vi "Preferences.vi"() -> ()   [LabVIEW 2014]
uses:
  globals/AzCamGlobals.vi
panel:
  in  "Enable Telescope":bool
  in  "Enable Instrument":bool
  in  "ShowClientCommands":bool caption="Show client commands"
  in  "SequenceFlushing":enum32{"All", "Once", "None"}(radio)
  in  "Sequence\nDelay (secs)":dbl format="%#.3g"
  in  "ReadTemps":bool caption="Read temperatures"
  in  "Reload":bool
  in  "AutoTitle":bool caption="Auto title images"
  in  "ShowUserWarnings":bool=TRUE caption="Show User Warnings"
  in  "Use Sound":bool
  in  "Prompt4Title":bool caption="Prompt for Image Title"
  in  "ClearArray":bool=TRUE caption="Clear Array before each exposure"
  in  "Display image":bool=TRUE
  in  "Image Header File":path=path "NONE"
  in  "EditHeaderFile":bool
  in  "Exit":bool
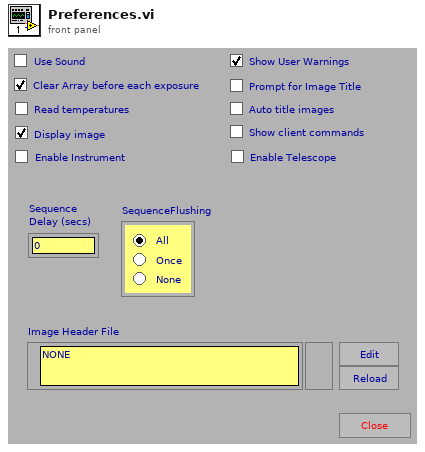
[diagram p1: front panel]
types:
  T1 = enum16{"Status", "CamTemp", "DewTemp", "GetExpose", "GetSequence", "SetExpose", "Filename", "ColBin", "RowBin"}
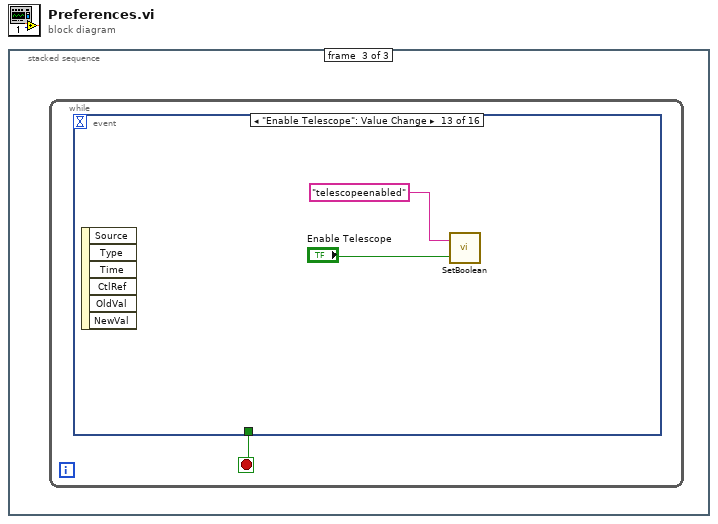
[diagram p0: block diagram]
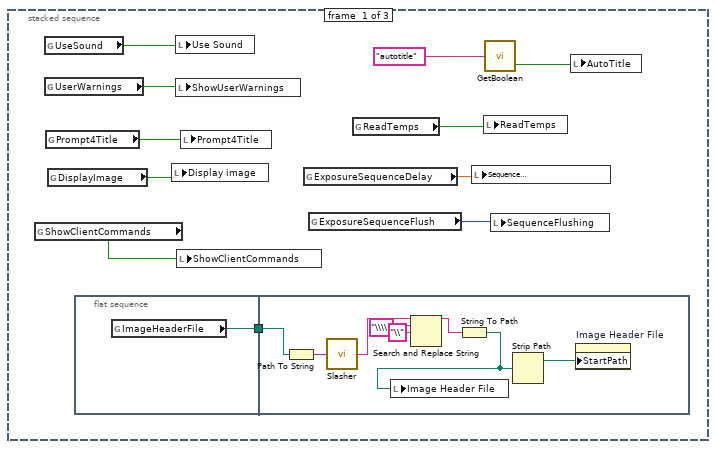
[diagram p2: hidden frame]
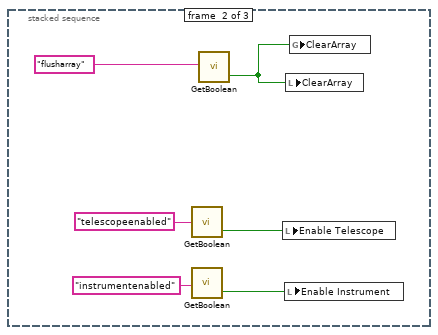
[diagram p3: hidden frame]
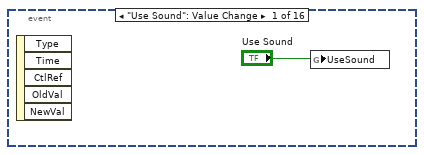
[diagram p4: hidden frame]
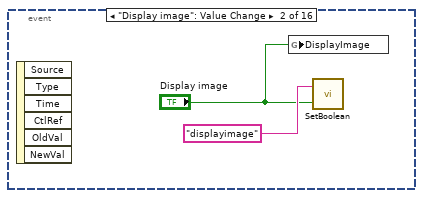
[diagram p5: hidden frame]
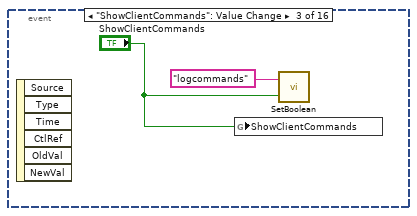
[diagram p6: hidden frame]
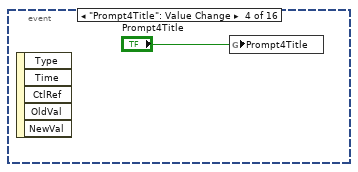
[diagram p7: hidden frame]
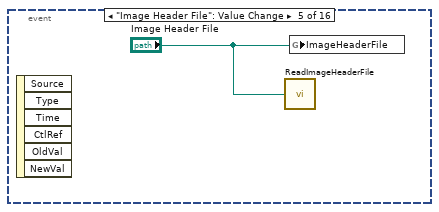
[diagram p8: hidden frame]
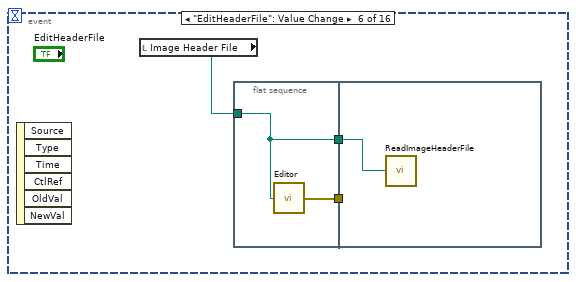
[diagram p9: hidden frame]
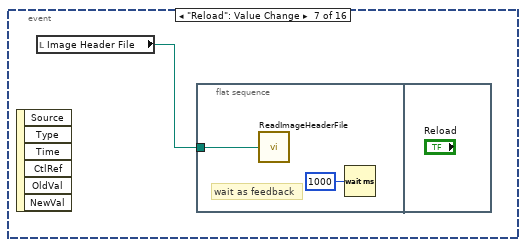
[diagram p10: hidden frame]
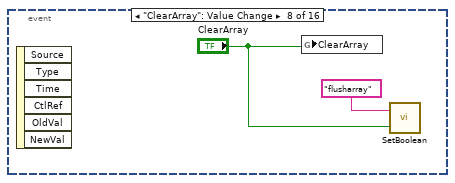
[diagram p11: hidden frame]
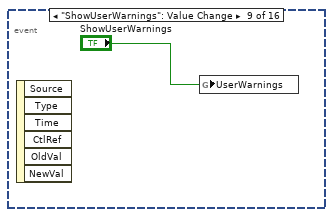
[diagram p12: hidden frame]
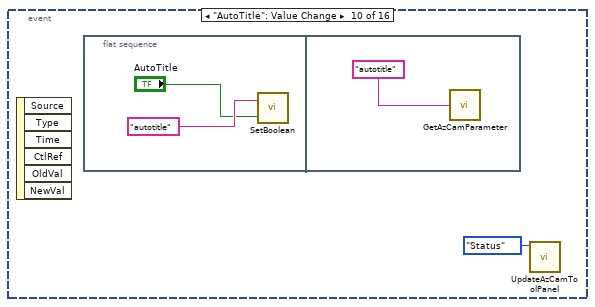
[diagram p13: hidden frame]
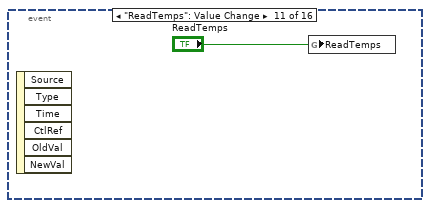
[diagram p14: hidden frame]
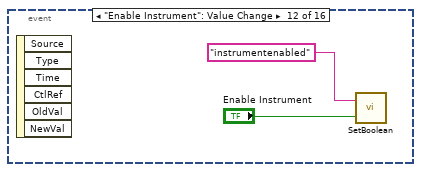
[diagram p15: hidden frame]
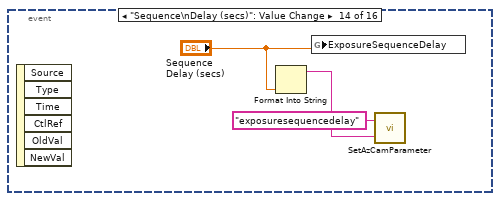
[diagram p16: hidden frame]
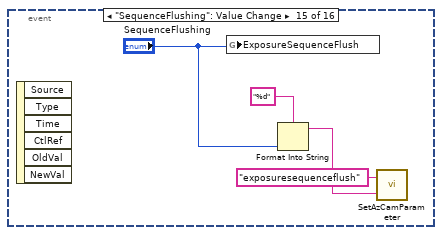
[diagram p17: hidden frame]
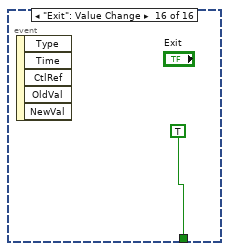
[diagram p18: hidden frame]
diagram:
  n1 = stacked-sequence {
    frame #0 {
      n2 = global read "AzCamGlobals.vi" "ShowClientCommands"() -> (w1:bool)
      n3 = global read "AzCamGlobals.vi" "UseSound"() -> (w7:bool)
      n4 = global read "AzCamGlobals.vi" "UserWarnings"() -> (w10:bool)
      n5 = global read "AzCamGlobals.vi" "Prompt4Title"() -> (w11:bool)
      n6 = global read "AzCamGlobals.vi" "DisplayImage"() -> (w3:bool)
      n7 = flat-sequence {
        tunnel: [w12] -> w2
        tunnel: w2 -> [w19]
        frame #0 {
          n8 = global read "AzCamGlobals.vi" "ImageHeaderFile"() -> (w12:path)
        }
        frame #1 {
          n9 = Path To String(path=w19) -> (string=w18:string)
          n10 = call "Slasher.vi"("String In"=w18) -> ("String Out"=w15:string)
          n11 = Search and Replace String(input string=w15, search string="\\\\" ("substring (\"\")"), replace string="\\" ("replace string (\"\")")) -> (result string=w14:string)  [unwired: 5 in, 3 out]
          n12 = String To Path(string=w14) -> (path=w13:path)
          n13 = local write "Image Header File"(w13) -> ()
          n14 = Strip Path(path=w13) -> (stripped path=w20:path)  [unwired: 1 out]
          n15 = property on="Image Header File" class="Path"("StartPath"=w20) -> ()  [unwired: 2 in, 2 out]
        }
      }
      n16 = local write "Display image"(w3) -> ()
      n17 = local write "Use Sound"(w7) -> ()
      n18 = local write "ShowUserWarnings"(w10) -> ()
      n19 = local write "ShowClientCommands"(w1) -> ()
      n20 = local write "Prompt4Title"(w11) -> ()
      n21 = global read "AzCamGlobals.vi" "ExposureSequenceDelay"() -> (w5:dbl)
      n22 = global read "AzCamGlobals.vi" "ExposureSequenceFlush"() -> (w4:i32)
      n23 = global read "AzCamGlobals.vi" "ReadTemps"() -> (w6:bool)
      n24 = local write "Sequence\nDelay (secs)"(w5) -> ()
      n25 = local write "ReadTemps"(w6) -> ()
      n26 = call "GetBoolean.vi"("Attribute"="autotitle") -> ("Boolean"=w8:bool)  [unwired: 1 out]
      n27 = local write "SequenceFlushing"(w4) -> ()
      n28 = local write "AutoTitle"(w8) -> ()
    }
    frame #1 {
      n29 = call "GetBoolean.vi"("Attribute"="telescopeenabled") -> ("Boolean"=w21:bool)  [unwired: 1 out]
      n30 = call "GetBoolean.vi"("Attribute"="instrumentenabled" ("Command")) -> ("Boolean"=w22:bool)  [unwired: 1 out]
      n31 = call "GetBoolean.vi"("Attribute"="flusharray" ("Command")) -> ("Boolean"=w25:bool)  [unwired: 1 out]
      n32 = local write "Enable Telescope"(w21) -> ()
      n33 = local write "Enable Instrument"(w22) -> ()
      n34 = local write "ClearArray"(w25) -> ()
      n35 = global write "AzCamGlobals.vi" "ClearArray"(w25) -> ()
    }
    frame #2 {
      n36 = while {
        stop <- w27 stop-if-true
        n37 = event shown="[12] \"Enable Telescope\": Value Change" {
          selector: _ -> [_ _ _ _ _ _ _ _ _ _ _ _ _ _ _ _]
          dyn-events: _ -> [_ _ _ _ _ _ _ _ _ _ _ _ _ _ _ _]
          timeout: _ -> [_ _ _ _ _ _ _ _ _ _ _ _ _ _ _ _]
          tunnel: [_ _ _ _ _ _ _ _ _ _ _ _ _ _ _ TRUE] -> w27
          event "Use Sound": Value Change {
            n38 = event-data() -> ()  [unwired: 1 in, 5 out]
            n39 = global write "AzCamGlobals.vi" "UseSound"("Use Sound") -> ()
          }
          event "Display image": Value Change {
            n40 = event-data() -> ()  [unwired: 1 in, 6 out]
            n41 = global write "AzCamGlobals.vi" "DisplayImage"("Display image") -> ()
            n42 = call "SetBoolean.vi"("Boolean"="Display image", "Attribute"="displayimage" ("Command")) -> ()  [unwired: 1 out]
          }
          event "ShowClientCommands": Value Change {
            n43 = event-data() -> ()  [unwired: 1 in, 6 out]
            n44 = global write "AzCamGlobals.vi" "ShowClientCommands"("ShowClientCommands") -> ()
            n45 = call "SetBoolean.vi"("Boolean"="ShowClientCommands", "Attribute"="logcommands" ("string")) -> ()  [unwired: 1 out]
          }
          event "Prompt4Title": Value Change {
            n46 = event-data() -> ()  [unwired: 1 in, 5 out]
            n47 = global write "AzCamGlobals.vi" "Prompt4Title"("Prompt4Title") -> ()
          }
          event "Image Header File": Value Change {
            n48 = event-data() -> ()  [unwired: 1 in, 6 out]
            n49 = call "ReadImageHeaderFile.vi"("ImageHeaderFile"="Image Header File") -> ()  [unwired: 1 in]
            n50 = global write "AzCamGlobals.vi" "ImageHeaderFile"("Image Header File") -> ()
          }
          event "EditHeaderFile": Value Change {
            n51 = event-data() -> ()  [unwired: 1 in, 6 out]
            n52 = local read "Image Header File"() -> (w37:path)
            n53 = flat-sequence {
              tunnel: w37 -> [w39]
              tunnel: [w39] -> w36
              tunnel: [w38] -> w35
              tunnel: w36 -> [w40]
              tunnel: w35 -> [_]
              frame #0 {
                n54 = call "Editor.vi"("File"=w39) -> ("error out"=w38:errorcluster)
              }
              frame #1 {
                n55 = call "ReadImageHeaderFile.vi"("ImageHeaderFile"=w40) -> ()  [unwired: 1 in]
              }
            }
          }
          event "Reload": Value Change {
            n56 = event-data() -> ()  [unwired: 1 in, 6 out]
            n57 = local read "Image Header File"() -> (w41:path)
            n58 = flat-sequence {
              tunnel: w41 -> [w43]
              frame #0 {
                # "wait as feedback"
                n59 = call "ReadImageHeaderFile.vi"("ImageHeaderFile"=w43) -> ()  [unwired: 1 in]
                n60 = Wait (ms)(milliseconds to wait=u32 1000) -> ()  [unwired: 1 out]
              }
              frame #1 {
              }
            }
          }
          event "ClearArray": Value Change {
            n61 = event-data() -> ()  [unwired: 1 in, 6 out]
            n62 = global write "AzCamGlobals.vi" "ClearArray"("ClearArray") -> ()
            n63 = call "SetBoolean.vi"("Boolean"="ClearArray", "Attribute"="flusharray" ("Command")) -> ()  [unwired: 1 out]
          }
          event "ShowUserWarnings": Value Change {
            n64 = event-data() -> ()  [unwired: 1 in, 6 out]
            n65 = global write "AzCamGlobals.vi" "UserWarnings"("ShowUserWarnings") -> ()
          }
          event "AutoTitle": Value Change {
            n66 = event-data() -> ()  [unwired: 1 in, 6 out]
            n67 = flat-sequence {
              frame #0 {
                n68 = call "SetBoolean.vi"("Boolean"="AutoTitle", "Attribute"="autotitle") -> ()  [unwired: 1 out]
              }
              frame #1 {
                n69 = call "GetAzCamParameter.vi"("Parameter"="autotitle" ("Command")) -> ()  [unwired: 2 out]
              }
            }
            n70 = call "UpdateAzCamToolPanel.vi"("Control"=T1."Status") -> ()  [unwired: 3 in, 1 out]
          }
          event "ReadTemps": Value Change {
            n71 = event-data() -> ()  [unwired: 1 in, 6 out]
            n72 = global write "AzCamGlobals.vi" "ReadTemps"("ReadTemps") -> ()
          }
          event "Enable Instrument": Value Change {
            n73 = event-data() -> ()  [unwired: 1 in, 6 out]
            n74 = call "SetBoolean.vi"("Boolean"="Enable Instrument", "Attribute"="instrumentenabled") -> ()  [unwired: 1 out]
          }
          event "Enable Telescope": Value Change {
            n75 = event-data() -> ()  [unwired: 1 in, 6 out]
            n76 = call "SetBoolean.vi"("Boolean"="Enable Telescope", "Attribute"="telescopeenabled") -> ()  [unwired: 1 out]
          }
          event "Sequence\nDelay (secs)": Value Change {
            n77 = event-data() -> ()  [unwired: 1 in, 6 out]
            n78 = Format Into String("Sequence\nDelay (secs)") -> (resulting string=w56:string)  [unwired: 3 in, 1 out]
            n79 = global write "AzCamGlobals.vi" "ExposureSequenceDelay"("Sequence\nDelay (secs)") -> ()
            n80 = call "SetAzCamParameter.vi"("Value"=w56, "Parameter"="exposuresequencedelay") -> ()  [unwired: 1 out]
          }
          event "SequenceFlushing": Value Change {
            n81 = event-data() -> ()  [unwired: 1 in, 6 out]
            n82 = global write "AzCamGlobals.vi" "ExposureSequenceFlush"("SequenceFlushing") -> ()
            n83 = Format Into String(format string="%d", "SequenceFlushing") -> (resulting string=w59:string)  [unwired: 2 in, 1 out]
            n84 = call "SetAzCamParameter.vi"("Value"=w59, "Parameter"="exposuresequenceflush") -> ()  [unwired: 1 out]
          }
          event "Exit": Value Change {
            n85 = event-data() -> ()  [unwired: 1 in, 5 out]
          }
        }
      }
    }
  }
